vi "TCI.vi"(7 "codo arriba":bool, 8 "theta2Actual":dbl, 9 "py":dbl, 10 "px":dbl, 11 "theta1Actual":dbl) -> (1 "theta2d":dbl, 2 "theta1d":dbl, 3 "fueraEspacioDeTrabajo":bool)   [LabVIEW 2019]
panel:
  out "theta2":dbl
  out "theta1":dbl
  out "betha":dbl
  out "alpha":dbl
  out "gamma":dbl
  out "LT":dbl
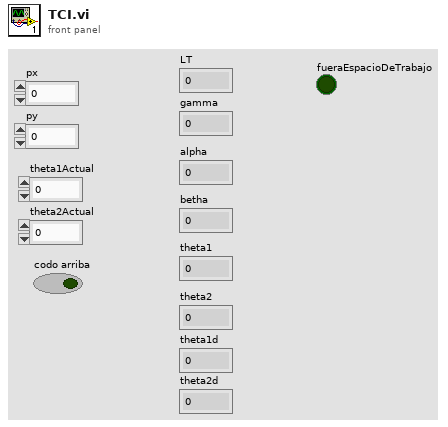
[diagram p1: front panel]
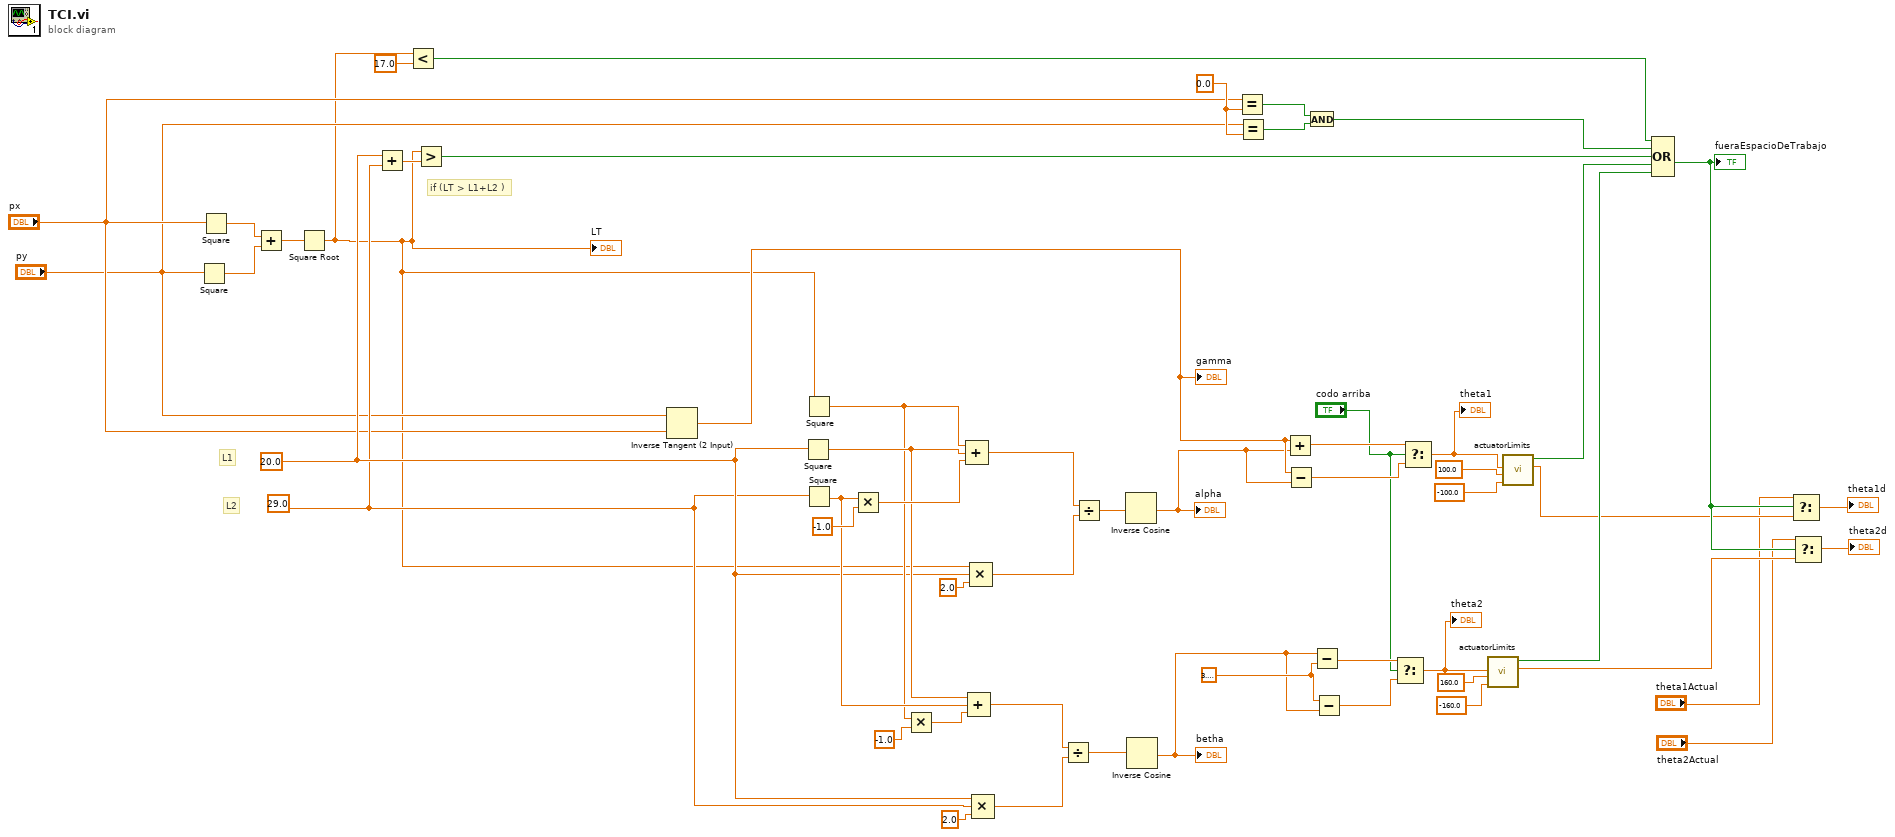
[diagram p0: block diagram]
diagram:
  w9 = 0.0 ("y")
  w26 = 29.0 ("x")
  w27 = 20.0 ("x")
  w31 = 3.141592653589793
  # "if (LT > L1+L2 )"
  # "L2"
  # "L1"
  n1 = Square(x="py") -> (x^2=w54:dbl)
  n2 = Square(x="px") -> (x^2=w55:dbl)
  n3 = Add(x=w55, y=w54) -> (x+y=w53:dbl)
  n4 = Square Root(x=w53) -> (sqrt(x)=w3:dbl)
  "LT" <- w3
  n5 = Add(x=w27, y=w26) -> (x+y=w28:dbl)
  n6 = Less?(x=w3, y=17.0) -> (x < y?=w1:bool)
  n7 = Greater?(x=w3, y=w28) -> (0:w21:bool)
  n8 = Inverse Tangent (2 Input)(1:"px", 2:"py") -> (0:w35:dbl)
  "gamma" <- w35
  n9 = Square(x=w27) -> (x^2=w46:dbl)
  n10 = Square(x=w3) -> (x^2=w42:dbl)
  n11 = Square(x=w26) -> (x^2=w45:dbl)
  n12 = Multiply(x=w45, y=-1.0) -> (x*y=w51:dbl)
  n13 = Multiply(x=w42, y=-1.0) -> (x*y=w43:dbl)
  n14 = Compound Arithmetic op=ADD(w42, w46, w51) -> (w49:dbl)
  n15 = Compound Arithmetic op=ADD(w46, w45, w43) -> (w39:dbl)
  n16 = Compound Arithmetic op=MULTIPLY(w3, w27, 2.0 ("value")) -> (w48:dbl)
  n17 = Compound Arithmetic op=MULTIPLY(w27, w26, 2.0 ("value")) -> (w40:dbl)
  n18 = Divide(x=w39, y=w40) -> (x/y=w38:dbl)
  n19 = Divide(x=w49, y=w48) -> (x/y=w47:dbl)
  n20 = Inverse Cosine(1:w47) -> (0:w34:dbl)
  "alpha" <- w34
  n21 = Inverse Cosine(1:w38) -> (0:w30:dbl)
  "betha" <- w30
  n22 = Equal?(x="px", y=w9) -> (x = y?=w8:bool)
  n23 = Equal?(x="py", y=w9) -> (x = y?=w7:bool)
  n24 = Add(x=w35, y=w34) -> (x+y=w37:dbl)
  n25 = Subtract(x=w35, y=w34) -> (x-y=w36:dbl)
  n26 = And(x=w8, y=w7) -> (x .and. y?=w6:bool)
  n27 = Subtract(x=w30, y=w31) -> (x-y=w33:dbl)
  n28 = Subtract(x=w31, y=w30) -> (x-y=w29:dbl)
  n29 = Select(t=w33, s="codo arriba", f=w29) -> (s? t:f=w17:dbl)
  "theta2" <- w17
  n30 = Select(t=w37, s="codo arriba", f=w36) -> (s? t:f=w18:dbl)
  "theta1" <- w18
  n31 = call "actuatorLimits.vi"("valorMinimo"=-160.0 ("y"), "valorMaximo"=160.0 ("y"), "valorEntrada"=w17) -> ("valorSalida"=w12:dbl, "fueraDelEspacioDeTrabajo"=w19:bool)  [unwired: 7 in]
  n32 = call "actuatorLimits.vi"("valorMinimo"=-100.0 ("y"), "valorMaximo"=100.0 ("y"), "valorEntrada"=w18) -> ("valorSalida"=w13:dbl, "fueraDelEspacioDeTrabajo"=w20:bool)  [unwired: 7 in]
  n33 = Compound Arithmetic op=OR(w1, w6, w21, w20, w19) -> (w14:bool)
  "fueraEspacioDeTrabajo" <- w14
  n34 = Select(t="theta1Actual", s=w14, f=w13) -> (s? t:f=→"theta1d":dbl)
  n35 = Select(t="theta2Actual", s=w14, f=w12) -> (s? t:f=→"theta2d":dbl)
